vi "TDMSLogger_PowerScan_Init.vi"(0 "object in":refnum<class "TDMSLogger_PowerScan.lvclass">, 5 "error in (no error)":errorcluster) -> (14 "object out":refnum<class "TDMSLogger_PowerScan.lvclass">, 16 "cancelled":bool, 19 "error out":errorcluster)   [LabVIEW 2023, in "TDMSLogger_PowerScan.lvclass"]
uses:
  TDMSLogger_PowerScan.lvclass
  TDMSLogger_PowerScan.lvclass/TDMSLogger_PowerScan.ctl
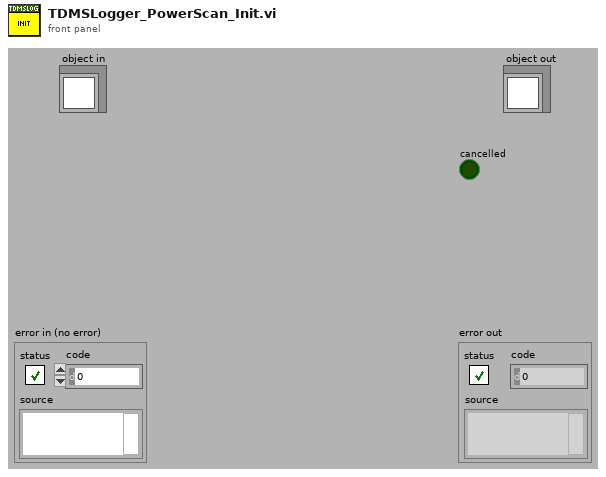
[diagram p1: front panel]
types:
  T1 = enum16{"open", "open or create", "create or replace", "create", "open (read-only)"}
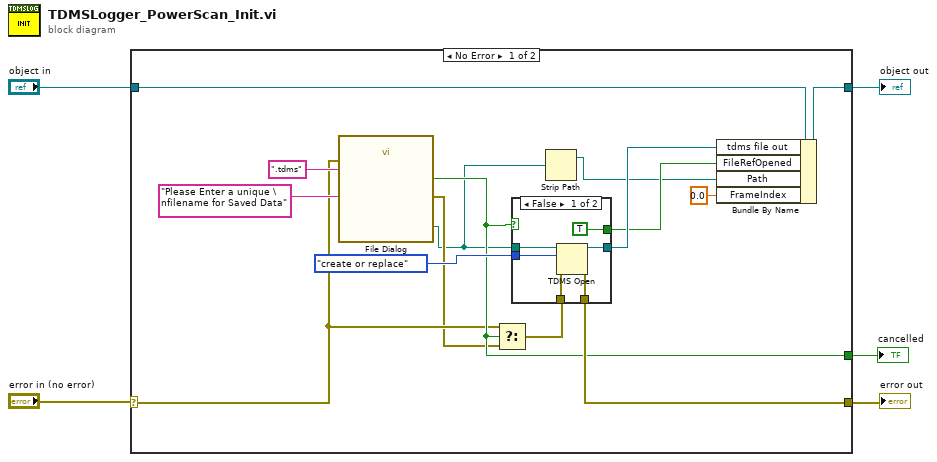
[diagram p0: block diagram]
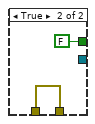
[diagram p2: hidden frame]
diagram:
  n1 = case shown="No Error" "error in (no error)" {
    selector: "error in (no error)" -> [w11 w29]
    tunnel: "object in" -> [w20 w30]
    tunnel: [w19 w30] -> w4
    tunnel: [w18 w29] -> w2
    tunnel: [w12 _] -> w1
    frame No Error {
      n2 = call "File Dialog"("prompt"="Please Enter a unique \nfilename for Saved Data", "error in"=w11, "pattern (all files)"=".tdms") -> ("selected path"=w8:path, "cancelled"=w12:bool, "error out"=w10:errorcluster)  [unwired: 9 in, 1 out]
      n3 = Select(t=w11, s=w12, f=w10) -> (s? t:f=w9:errorcluster)
      n4 = case shown="False" w12 {
        tunnel: [w26 w28] -> w18
        tunnel: w8 -> [w25 _]
        tunnel: [w24 _] -> w17
        tunnel: T1."create or replace" ("operation (0:open)") -> [w23 _]
        tunnel: w9 -> [w22 w28]
        tunnel: [TRUE FALSE] -> w13
        frame False {
          n5 = TDMS Open(8:w22, 10:w23, 11:w25) -> (0:w26:errorcluster, 3:w24:refnum<k34>)  [unwired: 4 in]
        }
        frame True {
        }
      }
      n6 = Strip Path(path=w8) -> (stripped path=w7:path)  [unwired: 1 out]
      n7 = Bundle By Name(cluster=w20, "tdms file out"=w17, "FileRefOpened"=w13, "Path"=w7, "FrameIndex"=0.0) -> (w19:refnum<class "TDMSLogger_PowerScan.lvclass">)
    }
    frame Error {
    }
  }
  "object out" <- w4
  "error out" <- w2
  "cancelled" <- w1
